vi "loadCRHSocketReport.vi"() -> ()   [LabVIEW 2012]
uses:
  <vilib>/addons/database/Connection.llb/DB Tools Open Connec (Path).vi
  <vilib>/addons/database/Connection.llb/Conn Execute.vi
  <vilib>/addons/database/Recordset.llb/Rec Destroy - Connection.vi
  <vilib>/addons/database/NI_Database_API.lvlib
panel:
  in  "path":path=path "C:/temp/SocketReport"
  out "before substring":string
  out "String":string
  out "after substring 2":string
  out "after substring":string
  out "array":string[][](array[string])
  out "concatenated string":string
  out "error out":errorcluster
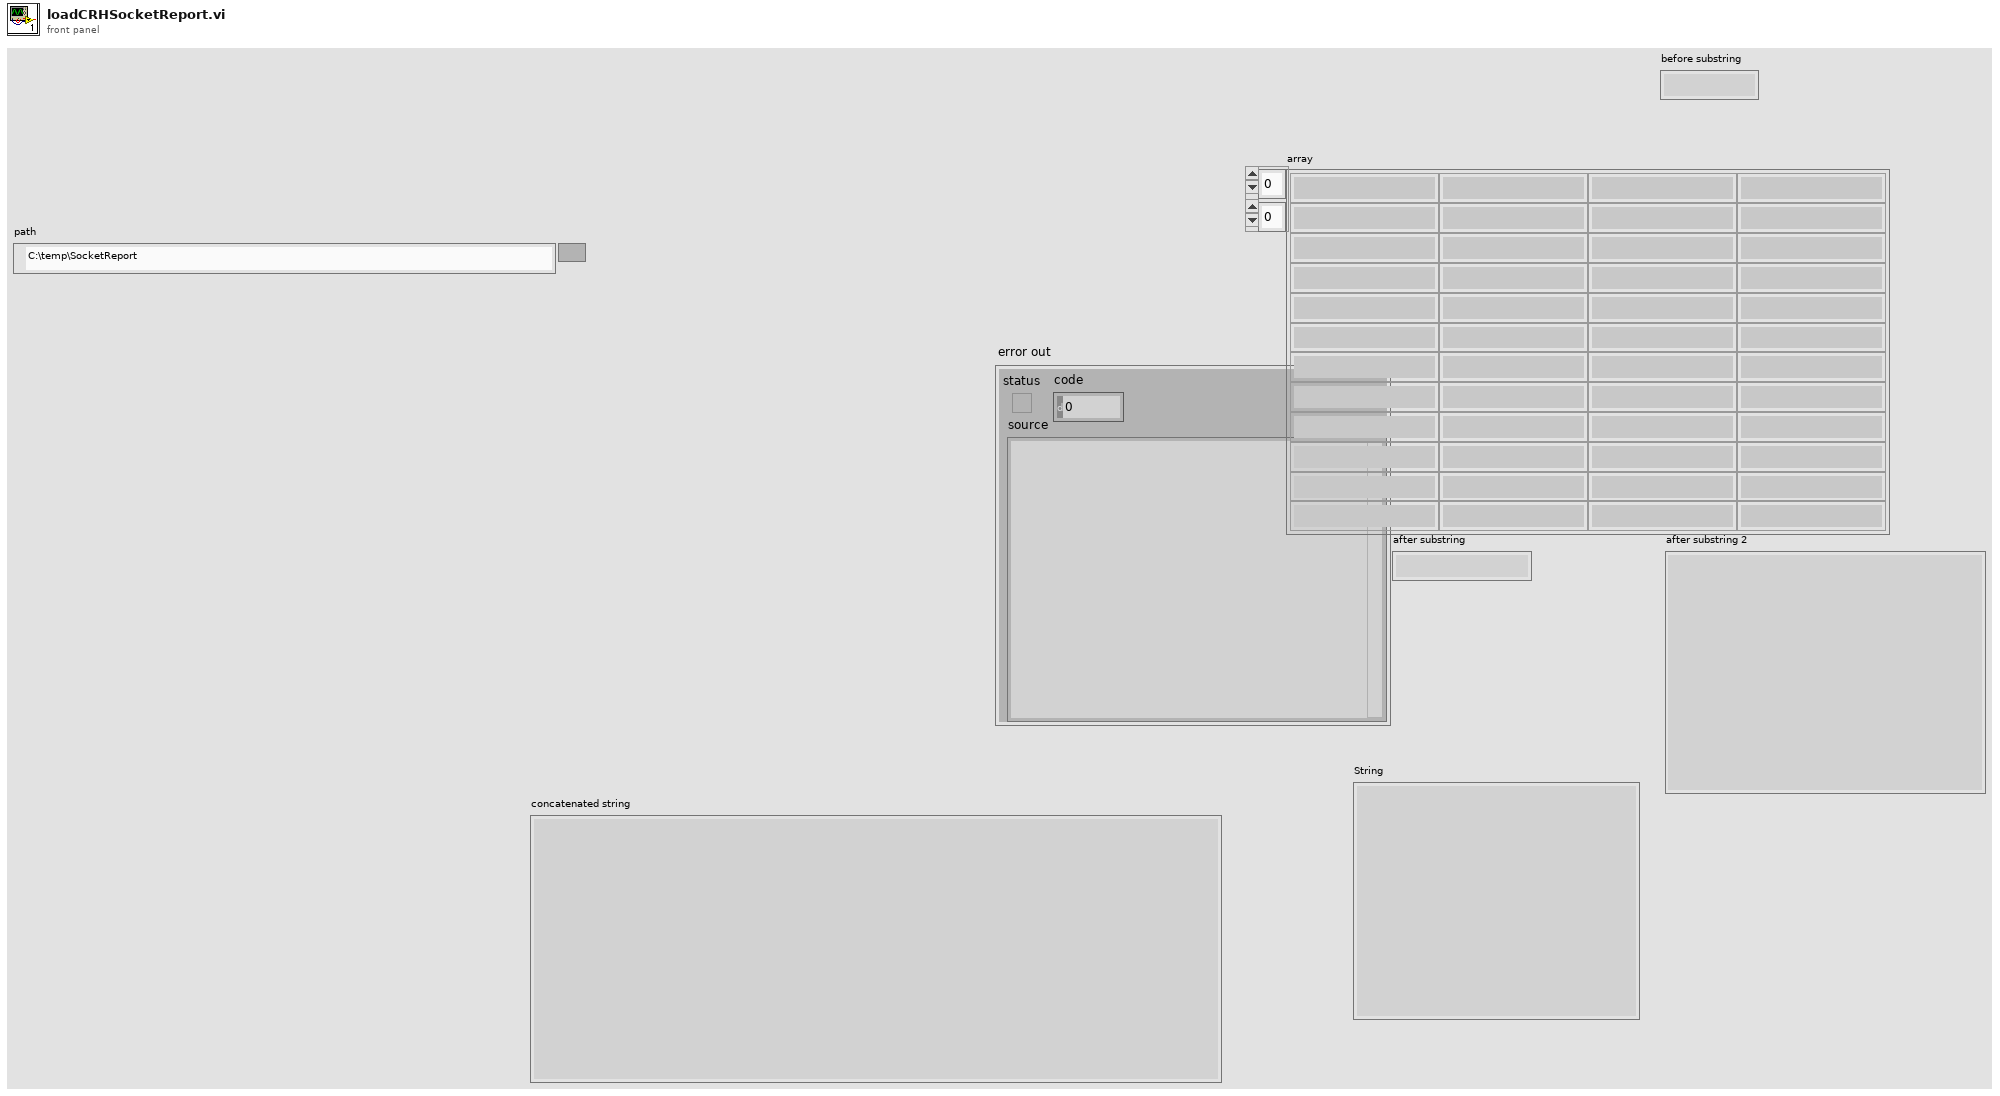
[diagram p1: front panel]
types:
  T1 = typedef "NI_Database_API.lvlib/Conn ObjectReference.ctl" = refnum<k1>
  T2 = typedef "NI_Database_API.lvlib/Rec ObjectReference.ctl" = refnum<k1>
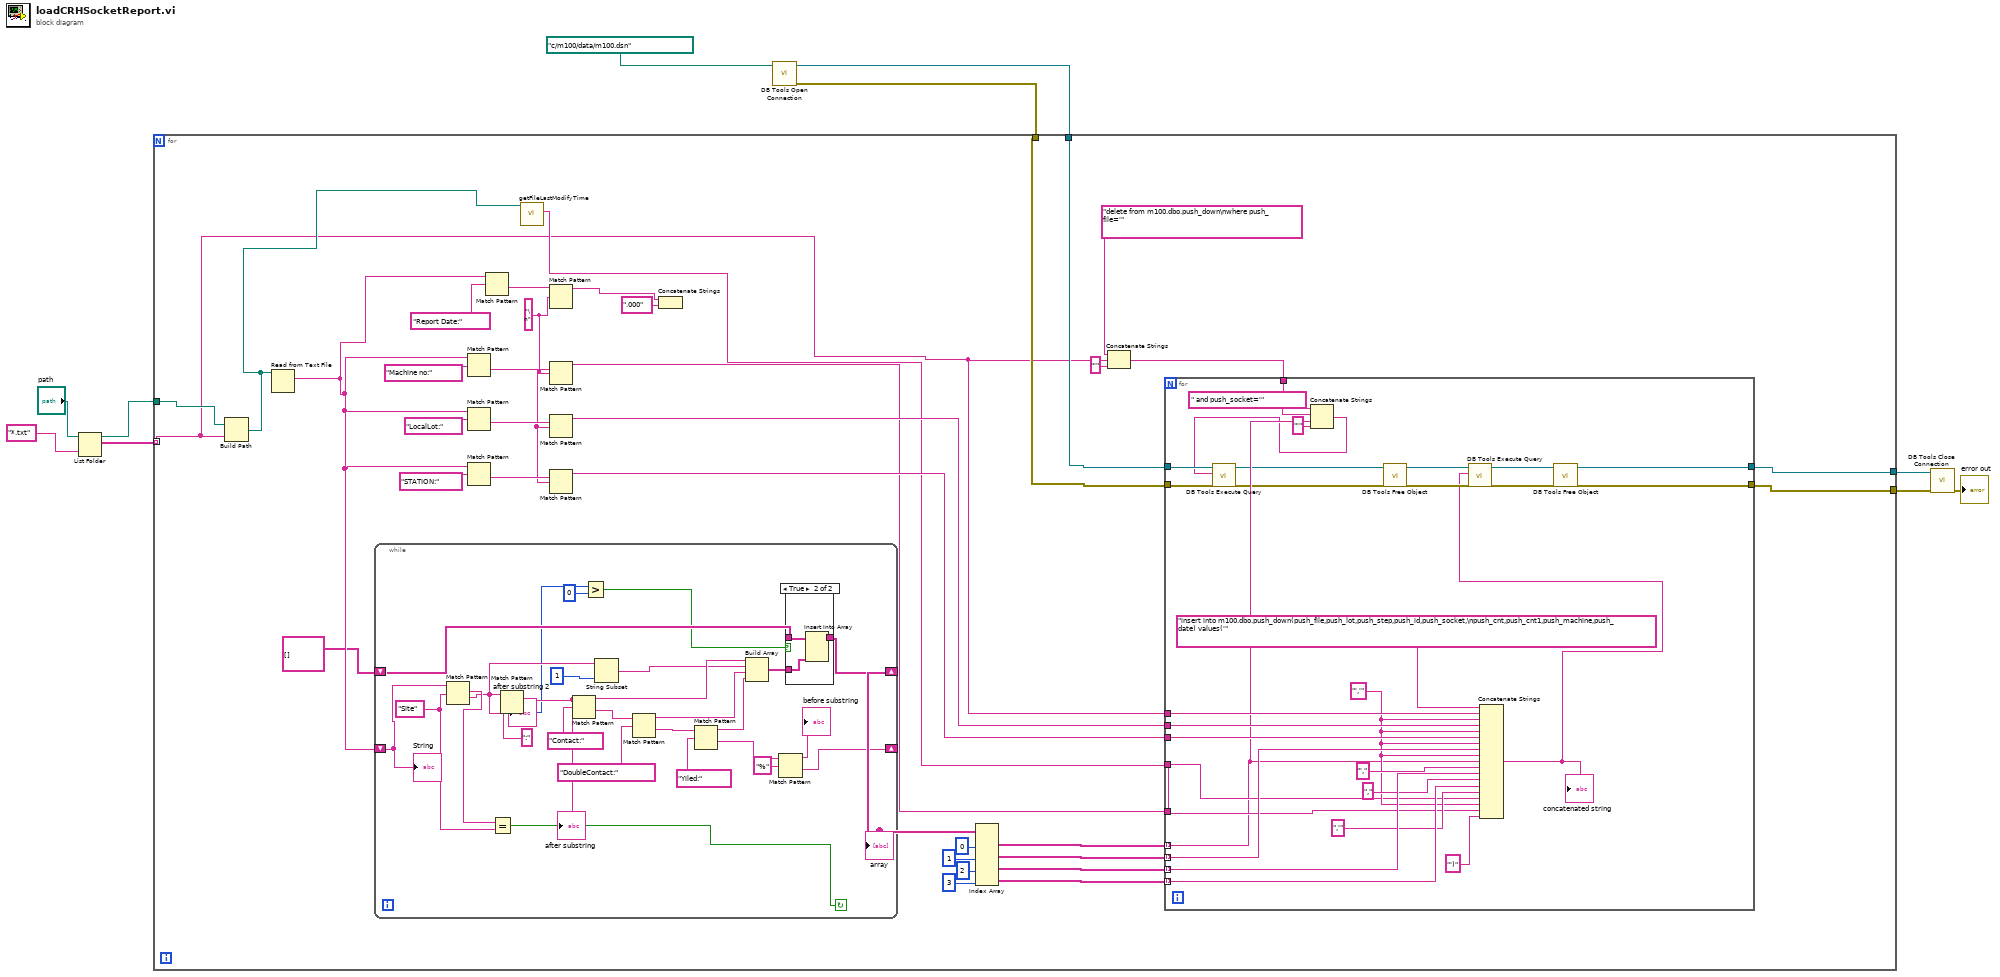
[diagram p0: block diagram]
diagram:
  n1 = List Folder(path="path", pattern="*.txt") -> (path out=w8:path, filenames=w1:string[])  [unwired: 2 in, 2 out]
  n2 = call-poly <vilib>:"DB Tools Open Connection.vi"("connection information"=path "c:/m100/data/m100.dsn") -> ("error out"=w2:errorcluster, "connection reference"=w3:T1)  [unwired: 7 in]
  n3 = for {
    tunnel: w8 -> [w13]
    tunnel: [w17] -> w6
    tunnel: [w16] -> w5
    tunnel: w3 -> [w15]
    tunnel: w2 -> [w14]
    tunnel: w1 -> [w11] mode=indexing
    w36 = "\n" ("regular expression")
    n4 = Build Path(base path=w13, name or relative path=w11) -> (appended path=w12:path)
    n5 = Read from Text File(file (use dialog)=w12) -> (text=w21:string)  [unwired: 3 in, 3 out]
    n6 = while {
      shift-right: [w49] -> _
      shift-left: w21 -> [w62]
      shift-right: [w61] -> w19
      shift-left: string[][] [] ("array") -> [w60]
      stop <- w57 continue-if-true
      w58 = "Site" ("regular expression")
      n7 = Match Pattern(string=w62, regular expression=w58) -> (match substring=w59:string, after substring=w54:string)  [unwired: 1 in, 2 out]
      "after substring 2" <- w54
      n8 = Equal?(x=w59, y=w58) -> (x = y?=w57:bool)
      n9 = Match Pattern(string=w54, regular expression=":") -> (after substring=w56:string, offset past match=w53:i32)  [unwired: 1 in, 2 out]
      "after substring" <- w56
      n10 = Match Pattern(string=w56, regular expression="Contact:") -> (before substring=w72:string, after substring=w70:string)  [unwired: 1 in, 2 out]
      n11 = Greater?(x=w53, y=0) -> (0:w51:bool)
      n12 = String Subset(string=w54, length (rest)=1 ("length (rest)")) -> (substring=w63:string)  [unwired: 1 in]
      n13 = Match Pattern(string=w70, regular expression="DoubleContact:") -> (before substring=w66:string, after substring=w68:string)  [unwired: 1 in, 2 out]
      n14 = Match Pattern(string=w68, regular expression="Yiled:") -> (before substring=w65:string, after substring=w50:string)  [unwired: 1 in, 2 out]
      n15 = Build Array(w72, w63, w66, w65) -> (w71:string[])
      n16 = Match Pattern(string=w50, regular expression="%") -> (before substring=→"before substring":string, after substring=w49:string)  [unwired: 1 in, 2 out]
      n17 = case shown="True" w51 {
        tunnel: w71 -> [_ w77]
        tunnel: [w74 w76] -> w61
        tunnel: w60 -> [w74 w75]
        frame False {
        }
        frame True {
          n18 = Insert Into Array(array=w75, new element=w77) -> (w76:string[][])  [unwired: 2 in]
        }
      }
      "String" <- w62
    }
    "array" <- w19
    n19 = Match Pattern(string=w21, regular expression="Machine no:") -> (after substring=w45:string)  [unwired: 1 in, 3 out]
    n20 = Match Pattern(string=w21, regular expression="LocalLot:") -> (after substring=w39:string)  [unwired: 1 in, 3 out]
    n21 = Match Pattern(string=w21, regular expression="STATION:") -> (after substring=w37:string)  [unwired: 1 in, 3 out]
    n22 = Match Pattern(string=w21, regular expression="Report Date:") -> (after substring=w41:string)  [unwired: 1 in, 3 out]
    n23 = call "getFileLastModifyTime.vi"("path"=w12) -> ("date/time string"=w18:string)  [unwired: 10 in]
    n24 = Match Pattern(string=w41, regular expression=w36) -> (before substring=w24:string)  [unwired: 1 in, 3 out]
    n25 = Match Pattern(string=w45, regular expression=w36) -> (before substring=w22:string)  [unwired: 1 in, 3 out]
    n26 = Match Pattern(string=w39, regular expression=w36) -> (before substring=w32:string)  [unwired: 1 in, 3 out]
    n27 = Match Pattern(string=w37, regular expression=w36) -> (before substring=w31:string)  [unwired: 1 in, 3 out]
    n28 = Concatenate Strings(w24, ".000" ("string")) -> ()  [unwired: 1 out]
    n29 = Index Array(array=w19, index (col) #1=0 ("disabled index (col)"), index (col) #2=1 ("index (col)"), index (col) #3=2 ("index (col)"), index (col) #4=3 ("index (col)")) -> (element #1=w27:string[], element #2=w28:string[], element #3=w26:string[], element #4=w25:string[])  [unwired: 4 in]
    n30 = Concatenate Strings("delete from m100.dbo.push_down\nwhere push_file='", w11, "'" ("string")) -> (w33:string)
    n31 = for {
      tunnel: w15 -> [w107]
      tunnel: [w105] -> w17
      tunnel: w14 -> [w104]
      tunnel: [w102] -> w16
      tunnel: w33 -> [w87]
      tunnel: w11 -> [w100]
      tunnel: w32 -> [w99]
      tunnel: w31 -> [w98]
      tunnel: w28 -> [w97] mode=indexing
      tunnel: w27 -> [w85] mode=indexing
      tunnel: w26 -> [w95] mode=indexing
      tunnel: w25 -> [w93] mode=indexing
      tunnel: w18 -> [w90]
      tunnel: w22 -> [w88]
      w89 = "','" ("string")
      n32 = Concatenate Strings(w87, " and push_socket='" ("string"), w85, "'" ("string")) -> (w83:string)
      n33 = call-poly <vilib>:"DB Tools Execute Query.vi"("error in (no error)"=w104, "SQL query"=w83, "connection reference"=w107) -> ("error out"=w78:errorcluster, "recordset reference"=w79:T2)  [unwired: 5 in]
      n34 = call-poly <vilib>:"DB Tools Free Object.vi"("error in (no error)"=w78, "recordset reference"=w79) -> ("error out"=w103:errorcluster, "connection reference"=w106:T1)  [unwired: 8 in]
      n35 = Concatenate Strings("insert into m100.dbo.push_down(push_file,push_lot,push_step,push_id,push_socket,\npush_cnt,push_cnt1,push_machine,push_date) values('", w100, w89, w99, w89, w98, w89, w97, w89, w85, "'," ("string"), w95, "," ("string"), w93, ",'" ("string"), w88, w89, w90, "')" ("string")) -> (w82:string)
      "concatenated string" <- w82
      n36 = call-poly <vilib>:"DB Tools Execute Query.vi"("error in (no error)"=w103, "SQL query"=w82, "connection reference"=w106) -> ("error out"=w80:errorcluster, "recordset reference"=w81:T2)  [unwired: 5 in]
      n37 = call-poly <vilib>:"DB Tools Free Object.vi"("error in (no error)"=w80, "recordset reference"=w81) -> ("error out"=w102:errorcluster, "connection reference"=w105:T1)  [unwired: 8 in]
    }
  }
  n38 = call <vilib>:"DB Tools Close Connection.vi"("error in (no error)"=w5, "connection reference"=w6) -> ("error out"=→"error out":errorcluster)  [unwired: 5 in]
